vi "get_baidumap1.1.vi"() -> ()   [LabVIEW 2012]
uses:
  <vilib>/httpClient/POSTBuffer.vi
  <vilib>/httpClient/LabVIEWHTTPClient.lvlib
panel:
  out "Qpost":string
  in  "Boolean":bool
  out "error out":errorcluster
  out "map":refnum<user-event>
  in  "stop":bool
  in  "x":i32(slide)=12 scale=4.0..19.0
  in  "纬度":dbl format="%#_10g"
  in  "经度":dbl format="%#_10g"
  out "new picture":picture
  # "百度地图调用"
  # "V1.0"
  # "谷歌地图：39.9071185441,116.3743215955\n百度地图：39.9130635112,116.3808525539\n腾讯高德：39.9071109356,116.3743114471\n图吧地图：39.9065406756,116.3637110571\n谷歌地球：39.9057606756,116.3681310571\n北纬N39°54′20.74″ 东经E116°22′5.27″\n\n靠近：中国北京市北京市西城区西长安街\n周边：中国人保大厦 约145米"
  # "精准坐标定位查询"
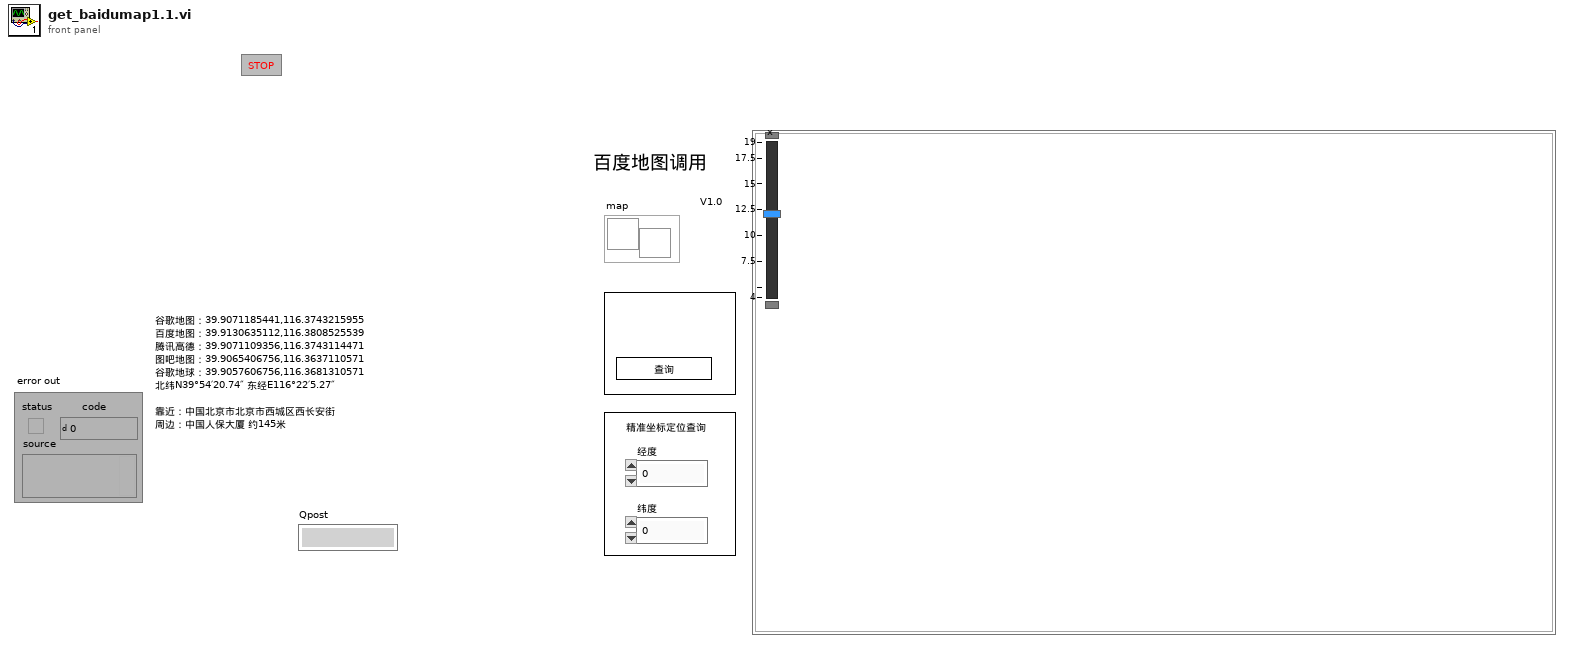
[diagram p1: front panel]
types:
  T1 = typedef "imagedata.ctl" = cluster{"image type":i32, "image depth":i32, "image":u8[], "mask":u8[], "colors":u32[], "Rectangle":cluster{"left":i16, "top":i16, "right":i16, "bottom":i16}}
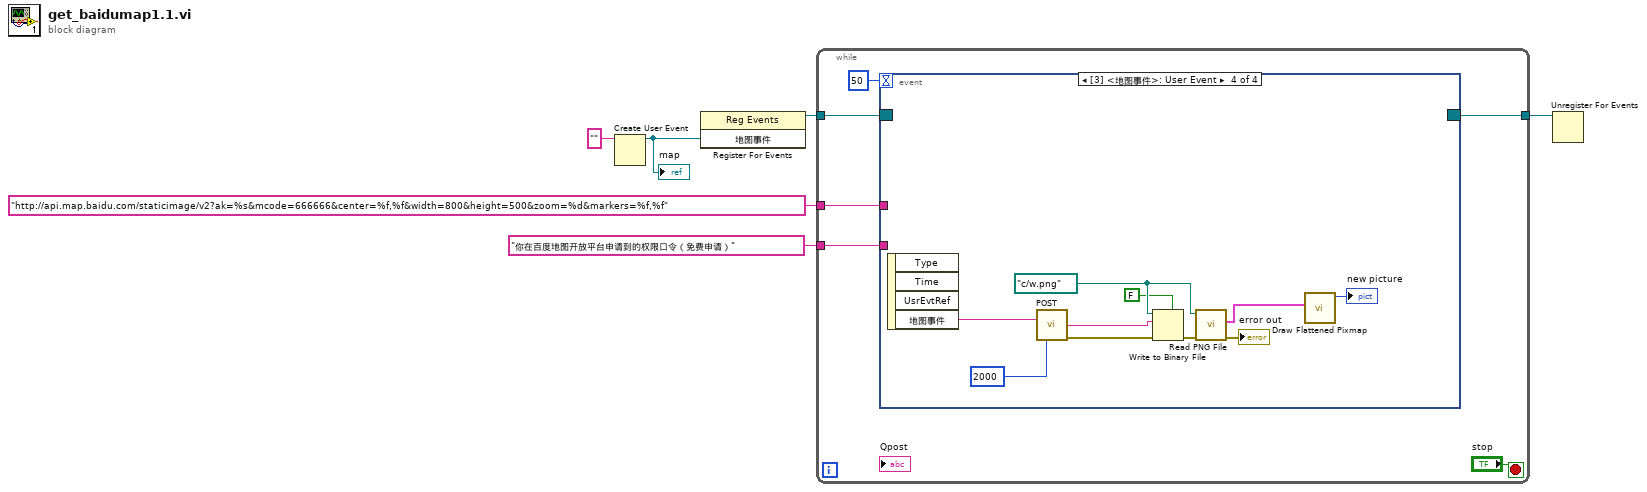
[diagram p0: block diagram]
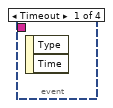
[diagram p2: hidden frame]
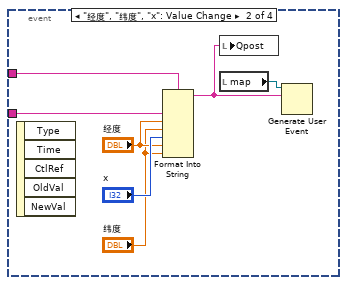
[diagram p3: hidden frame]
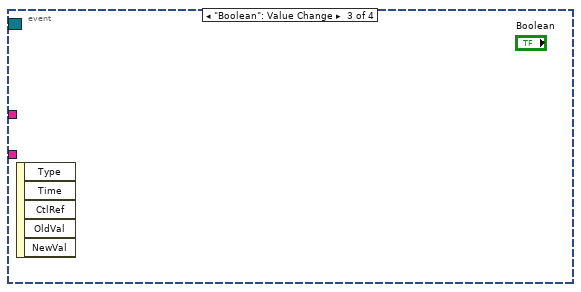
[diagram p4: hidden frame]
diagram:
  n1 = Create User Event(user event datatype="" ("地图事件")) -> (user event=w2:refnum<user-event>)  [unwired: 1 in, 1 out]
  "map" <- w2
  n2 = register-events(w2) -> (reference out=w5:refnum<event-registration>)  [unwired: 2 in, 1 out]
  n3 = while {
    tunnel: w5 -> [w11]
    tunnel: "http://api.map.baidu.com/staticimage/v2?ak=%s&mcode=666666&center=%f,%f&width=800&height=500&zoom=%d&markers=%f,%f" ("格式字符串") -> [w10]
    tunnel: [w8] -> w3
    tunnel: "你在百度地图开放平台申请到的权限口令（免费申请）" ("输入 1") -> [w7]
    stop <- "stop" stop-if-true
    n4 = event shown="[3] <地图事件>: User Event" {
      selector: w11 -> [_ _ _ _]
      dyn-events: [_ _ _ _] -> w8
      timeout: 50 -> [_ _ _ _]
      tunnel: w10 -> [_ w15 _ _]
      tunnel: w7 -> [_ w13 _ _]
      event Timeout {
        n5 = event-data() -> ()  [unwired: 1 in, 2 out]
      }
      event "经度", "纬度", "x": Value Change {
        n6 = event-data() -> ()  [unwired: 1 in, 5 out]
        n7 = Format Into String(format string=w15, w13, "经度", "纬度", "x", "经度", "纬度") -> (resulting string=w14:string)  [unwired: 2 in, 1 out]
        n8 = local write "Qpost"(w14) -> ()
        n9 = local read "map"() -> (w19:refnum<user-event>)
        n10 = Generate User Event(user event=w19, event data cluster=w14) -> ()  [unwired: 1 in, 2 out]
      }
      event "Boolean": Value Change {
        n11 = event-data() -> ()  [unwired: 1 in, 5 out]
      }
      event User Event {
        w28 = path "c:/w.png" ("file (use dialog)")
        n12 = event-data() -> ("地图事件"=w20:string)  [unwired: 1 in, 3 out]
        n13 = call-poly <vilib>:"POST.vi"("url"=w20, "timeout (10000)"=2000) -> ("body"=w25:string, "error out"=w22:errorcluster)  [unwired: 10 in, 2 out]
        n14 = Write to Binary File(file (use dialog)=w28, data=w25, error in=w22, 5:FALSE ("prepend array or string size? (T)")) -> (error out=w27:errorcluster)  [unwired: 2 in, 2 out]
        n15 = call <vilib>:"Read PNG File.vi"("error in (no error)"=w27, "path to PNG file"=w28) -> ("error out"=→"error out":errorcluster, "image data"=w29:T1)  [unwired: 7 in, 1 out]
        n16 = call <vilib>:"Draw Flattened Pixmap.vi"("image data"=w29) -> ("new picture"=→"new picture":picture)  [unwired: 8 in]
      }
    }
  }
  n17 = Unregister For Events(event registration refnum=w3) -> ()  [unwired: 1 in, 1 out]
